vi "USB2XXXIIC24C02.vi"() -> ()   [LabVIEW 2010]
panel:
  in  "接口电压":i8(ring)=3 items=["0 V", "1.8 V", "2.5 V", "3.3 V"]
  in  "pConfig":T1={"ClockSpeedHz"=100000, "OwnAddr"=0, "Master"=1, "AddrBits"=7, "EnablePu"=1}
  out "Read Data(Hex)":string
  in  "Read Data Count":i32=8
  in  "Reg Addr(Hex)":u8 format="%x"
  in  "Slave Addr(Hex)":i16=80 format="%x"
  in  "Write Data(Hex)":string="11 22 33 44 55 66 77 88"
  in  "Channel Index":i32(ring) items=["CH0", "CH1", "CH2", "CH3", "CH4", "CH5", "CH6", "CH7"]
  in  "Device Index":i32(ring) items=["0", "1", "2", "3", "4", "5"]
  out "Flag(T:Write;F:Read)":bool=TRUE
  in  "stop":bool
  in  "Read":bool
  in  "Write":bool
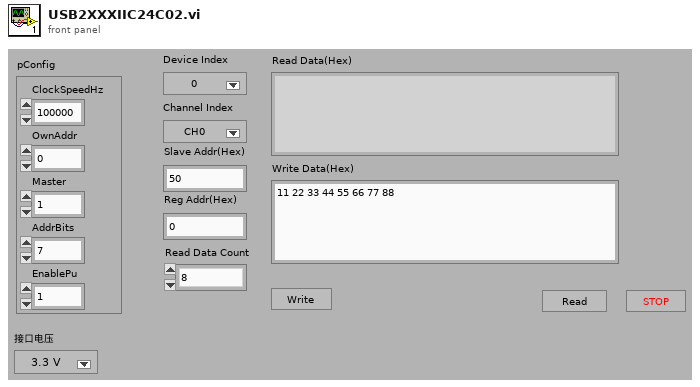
[diagram p1: front panel]
types:
  T1 = cluster{"ClockSpeedHz":u32, "OwnAddr":u16, "Master":u8, "AddrBits":u8, "EnablePu":u8}
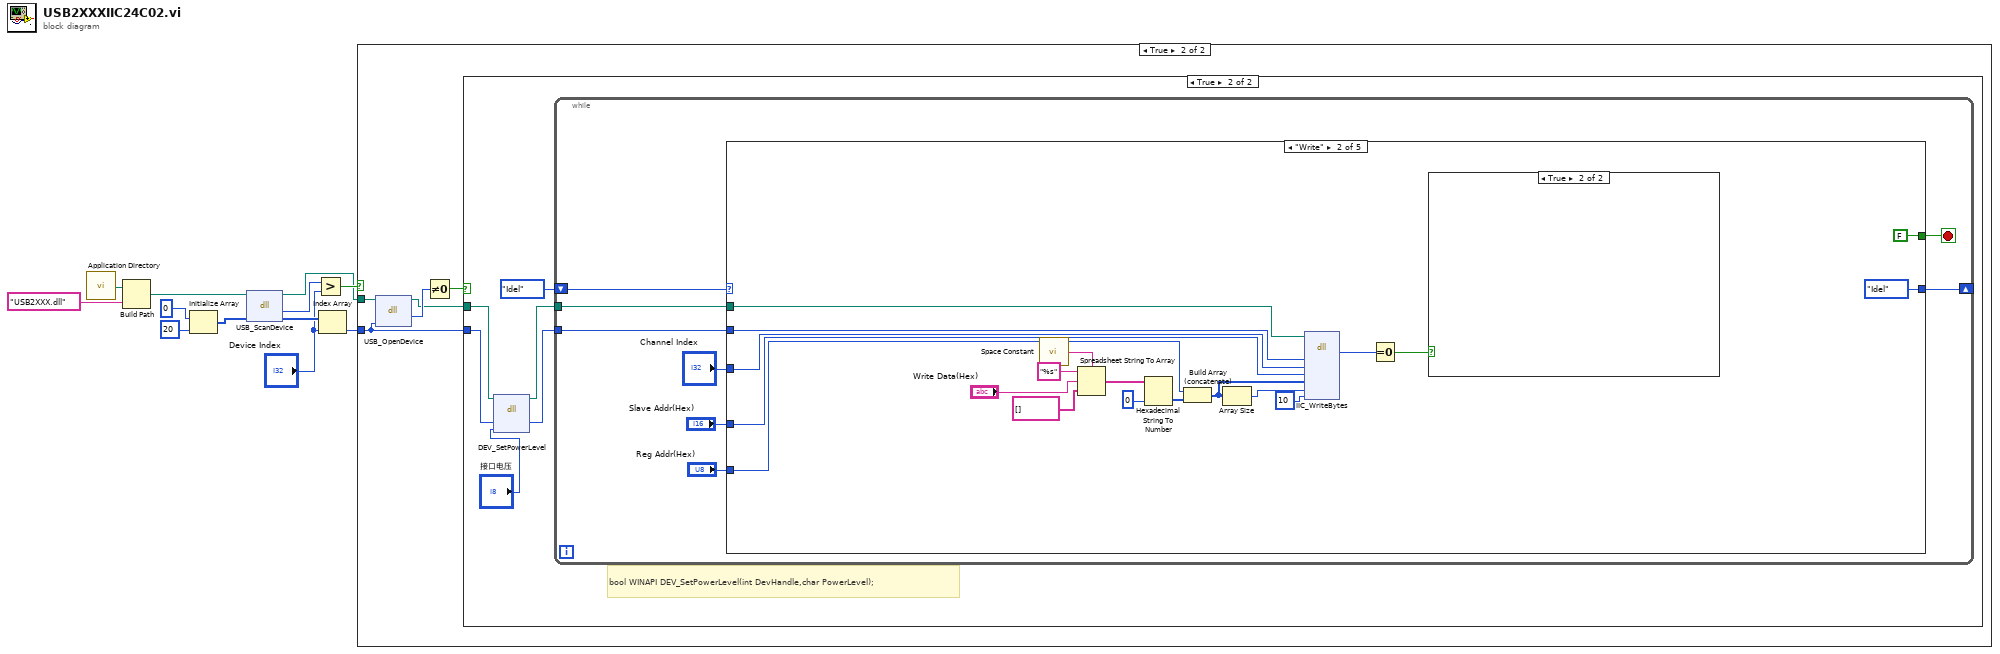
[diagram p0: block diagram]
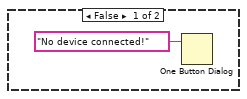
[diagram p2: hidden frame]
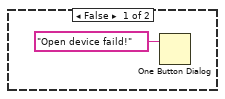
[diagram p3: hidden frame]
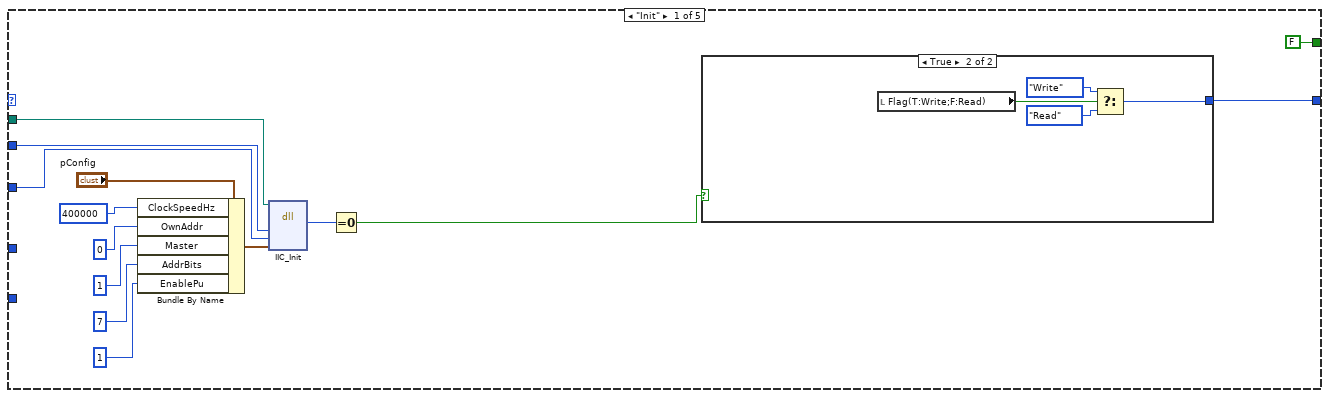
[diagram p4: hidden frame]
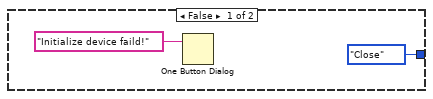
[diagram p5: hidden frame]
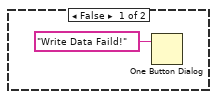
[diagram p6: hidden frame]
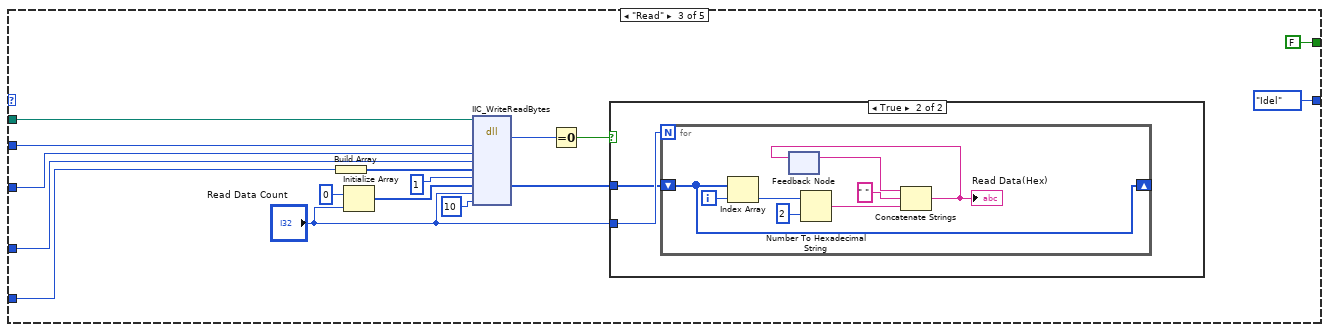
[diagram p7: hidden frame]
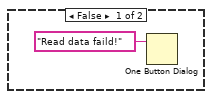
[diagram p8: hidden frame]
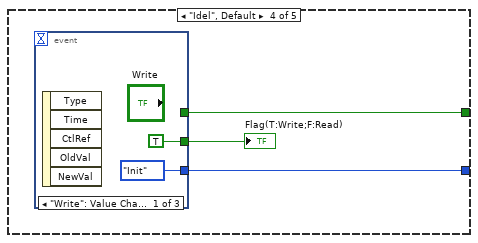
[diagram p9: hidden frame]
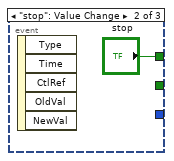
[diagram p10: hidden frame]
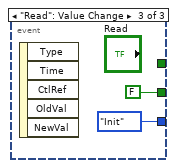
[diagram p11: hidden frame]
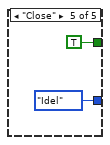
[diagram p12: hidden frame]
diagram:
  n1 = call <vilib>:"Application Directory.vi"() -> ("Application Directory"=w4:path)
  n2 = Build Path(base path=w4, name or relative path="USB2XXX.dll") -> (appended path=w3:path)
  n3 = Initialize Array(0, 20 ("dimension size")) -> (w9:i32[])
  n4 = dll-call lib="E:/Projects/USB2XXX_Example/sdk/api/Labview/USB2XXX.*" fn="USB_ScanDevice"(path in=w3, "pDevNum"=w9) -> (path out=w2:path, "return type"=w8:i32, "pDevNum"=w12:i32[])  [unwired: 2 in, 1 out]
  n5 = Greater?(x=w8, y="Device Index") -> (0:w7:bool)
  n6 = Index Array(array=w12, index="Device Index") -> (element=w6:i32)
  n7 = case shown="True" w7 {
    tunnel: w6 -> [_ w16]
    tunnel: w2 -> [_ w15]
    frame False {
      n8 = One Button Dialog(message="No device connected!") -> ()  [unwired: 1 in, 1 out]
    }
    frame True {
      n9 = dll-call lib="E:/Projects/USB2XXX_Example/sdk/api/Labview/USB2XXX.*" fn="USB_OpenDevice"(path in=w15, "DevIndex"=w16) -> (path out=w14:path, "return type"=w18:u8)  [unwired: 3 in, 1 out]
      n10 = Not Equal To 0?(x=w18) -> (x != 0?=w17:bool)
      n11 = case shown="True" w17 {
        tunnel: w16 -> [_ w22]
        tunnel: w14 -> [_ w24]
        frame False {
          n12 = One Button Dialog(message="Open device faild!") -> ()  [unwired: 1 in, 1 out]
        }
        frame True {
          # "bool WINAPI DEV_SetPowerLevel(int DevHandle,char PowerLevel);"
          n13 = dll-call lib="E:/Projects/USB2XXX/trunk/USB2XXX/USB2XXX/vs2010/Release/USB2XXX.*" fn="DEV_SetPowerLevel"(path in=w24, "DevHandle"=w22, "PowerLevel"="接口电压") -> (path out=w23:path, "DevHandle"=w21:i32)  [unwired: 4 in, 1 out]
          n14 = while {
            shift-right: [w32] -> _
            shift-left: enum16{"Init", "Write", "Read", "Idel", "Close"}."Idel" ("Enum") -> [w33]
            tunnel: w21 -> [w27]
            tunnel: w23 -> [w26]
            stop <- w28 stop-if-true
            n15 = case shown="\"Write\"" w33 {
              tunnel: [w35 enum16{"Init", "Write", "Read", "Idel", "Close"}."Idel" ("Enum") enum16{"Init", "Write", "Read", "Idel", "Close"}."Idel" ("Enum") w101 enum16{"Init", "Write", "Read", "Idel", "Close"}."Idel" ("Enum")] -> w32
              tunnel: "Channel Index" -> [w37 w66 w82 _ _]
              tunnel: "Slave Addr(Hex)" -> [_ w60 w83 _ _]
              tunnel: "Reg Addr(Hex)" -> [_ w59 w86 _ _]
              tunnel: [FALSE FALSE FALSE w102 TRUE] -> w28
              tunnel: w27 -> [w36 w56 w75 _ _]
              tunnel: w26 -> [w34 w54 w74 _ _]
              frame "Init" {
                n16 = Bundle By Name(cluster="pConfig", "ClockSpeedHz"=u32 400000, "OwnAddr"=u16 0, "Master"=u8 1, "AddrBits"=u8 7, "EnablePu"=u8 1) -> (w45:T1)
                n17 = dll-call lib="E:/Projects/USB2XXX_Example/sdk/api/Labview/USB2XXX.*" fn="IIC_Init"(path in=w34, "DevIndex"=w36, "IICIndex"=w37, "pConfig"=w45) -> ("return type"=w39:i32)  [unwired: 5 in, 2 out]
                n18 = Equal To 0?(x=w39) -> (x = 0?=w38:bool)
                n19 = case shown="True" w38 {
                  tunnel: [enum16{"Init", "Write", "Read", "Idel", "Close"}."Close" ("Enum") w50] -> w35
                  frame False {
                    n20 = One Button Dialog(message="Initialize device faild!") -> ()  [unwired: 1 in, 1 out]
                  }
                  frame True {
                    n21 = local read "Flag(T:Write;F:Read)"() -> (w53:bool)
                    n22 = Select(t=enum16{"Init", "Write", "Read", "Idel", "Close"}."Write" ("Enum"), s=w53, f=enum16{"Init", "Write", "Read", "Idel", "Close"}."Read" ("Enum")) -> (s? t:f=w50:enum16{"Init", "Write", "Read", "Idel", "Close"})
                  }
                }
              }
              frame "Write" {
                n23 = call <vilib>:"Space Constant.vi"() -> ("String"=w68:string)
                n24 = Spreadsheet String To Array(delimiter (Tab)=w68, format string="%s", spreadsheet string="Write Data(Hex)", array type (2D Dbl)=string[] []) -> (array=w71:string[])
                n25 = Hexadecimal String To Number(string=w71, default (0uL)=u8 0 ("default (0 U32)")) -> (number=w58:u8[])  [unwired: 1 in, 1 out]
                n26 = Build Array (concatenate)(w59, w58) -> (w55:u8[])
                n27 = Array Size(array=w55) -> (size(s)=w65:i32)
                n28 = dll-call lib="E:/Projects/USB2XXX_Example/sdk/api/Labview/USB2XXX.*" fn="IIC_WriteBytes"(path in=w54, "DevIndex"=w56, "IICIndex"=w66, "SlaveAddr"=w60, "pWriteData"=w55, "WriteLen"=w65, "TimeOutMs"=10) -> ("return type"=w63:i32)  [unwired: 8 in, 2 out]
                n29 = Equal To 0?(x=w63) -> (x = 0?=w62:bool)
                n30 = case shown="True" w62 {
                  frame False {
                    n31 = One Button Dialog(message="Write Data Faild!") -> ()  [unwired: 1 in, 1 out]
                  }
                  frame True {
                  }
                }
              }
              frame "Read" {
                n32 = Build Array(w86) -> (w84:u8[])
                n33 = Initialize Array(u8 0 ("element"), "Read Data Count") -> (w87:u8[])
                n34 = dll-call lib="E:/Projects/USB2XXX_Example/sdk/api/Labview/USB2XXX.*" fn="IIC_WriteReadBytes"(path in=w74, "DevIndex"=w75, "IICIndex"=w82, "SlaveAddr"=w83, "pWriteData"=w84, "WriteLen"=1 ("dimension size"), "pReadData"=w87, "ReadLen"="Read Data Count", "TimeOutMs"=10) -> ("return type"=w81:i32, "pReadData"=w77:u8[])  [unwired: 9 in, 2 out]
                n35 = Equal To 0?(x=w81) -> (x = 0?=w80:bool)
                n36 = case shown="True" w80 {
                  tunnel: "Read Data Count" -> [_ w92]
                  tunnel: w77 -> [_ w91]
                  frame False {
                    n37 = One Button Dialog(message="Read data faild!") -> ()  [unwired: 1 in, 1 out]
                  }
                  frame True {
                    n38 = for {
                      N: w92 -> [_]
                      shift-right: [w93] -> _
                      shift-left: w91 -> [w93]
                      i -> [w100]
                      n39 = Index Array(array=w93, index=w100) -> (element=w99:u8)
                      n40 = feedback #1() -> (w97:string)  [unwired: 1 in]
                      n41 = Number To Hexadecimal String(1:i16 2 ("width (-)"), 2:w99) -> (0:w95:string)
                      n42 = Concatenate Strings(w97, " " ("string"), w95) -> (w94:string)
                      "Read Data(Hex)" <- w94
                      n43 = feedback-in #1(w94) -> ()
                    }
                  }
                }
              }
              frame "Idel", Default {
                n44 = event shown="[0] \"Write\": Value Change" {
                  selector: _ -> [_ _ _]
                  dyn-events: _ -> [_ _ _]
                  timeout: _ -> [_ _ _]
                  tunnel: [TRUE _ FALSE] -> w103
                  tunnel: [_ "stop" _] -> w102
                  tunnel: [enum16{"Init", "Write", "Read", "Idel", "Close"}."Init" ("Enum") _ enum16{"Init", "Write", "Read", "Idel", "Close"}."Init" ("Enum")] -> w101
                  event "Write": Value Change {
                    n45 = event-data() -> ()  [unwired: 1 in, 5 out]
                  }
                  event "stop": Value Change {
                    n46 = event-data() -> ()  [unwired: 1 in, 5 out]
                  }
                  event "Read": Value Change {
                    n47 = event-data() -> ()  [unwired: 1 in, 5 out]
                  }
                }
                "Flag(T:Write;F:Read)" <- w103
              }
              frame "Close" {
              }
            }
          }
        }
      }
    }
  }
